vi "DDS.vi"() -> ()   [LabVIEW 2021]
uses:
  <vilib>/RTI DDS Toolkit/Types/RTI DDS Advanced Writer Configuration.ctl
  <vilib>/RTI DDS Toolkit/Types/RTI DDS Advanced Reader Configuration.ctl
  <vilib>/Platform/TimedLoop/XDataNode/timing_clust.ctl
  <vilib>/Platform/TimedLoop/XDataNode/nitl_modes.ctl
  <vilib>/Platform/TimedLoop/XDataNode/wakeup.ctl
  <vilib>/RTI DDS Toolkit/VIs/AdvancedCreateWriter_NumI32.vi
  <vilib>/RTI DDS Toolkit/VIs/Write_NumI32.vi
  <vilib>/Platform/TimedLoop/XDataNode/XDataNode.xnode
  <vilib>/RTI DDS Toolkit/VIs/Read_NumI32.vi
  <vilib>/RTI DDS Toolkit/VIs/AdvancedCreateReader_NumI32.vi
  <vilib>/RTI DDS Toolkit/Library/LVDDS_library.lvlib
  <vilib>/Platform/TimedLoop/XDataNode/XDNodeRunTimeDep.lvlib
panel:
  in  "Advanced Reader Configuration":T1={"typeName"="std_msgs::msg::dds_::Int32_", "keyName"="", "domainParticipantQoSProfile"="", "dataReaderQoSProfile"="", "forceArrayMapping?"=FALSE, "forceExclusiveReader?"=FALSE, "forceRead? (only ExclusiveReader)"=FALSE, "forceUnboundedString?"=FALSE}
  in  "error in (no error)":errorcluster
  in  "Advanced Writer Configuration":T2={"typeName"="std_msgs::msg::dds_::Int32_", "keyName"="", "domainParticipantQoSProfile"="", "dataWriterQoSProfile"="", "forceArrayMapping?"=FALSE, "forceUnboundedString?"=FALSE}
  in  "stop":bool
  # "DDS Communication"
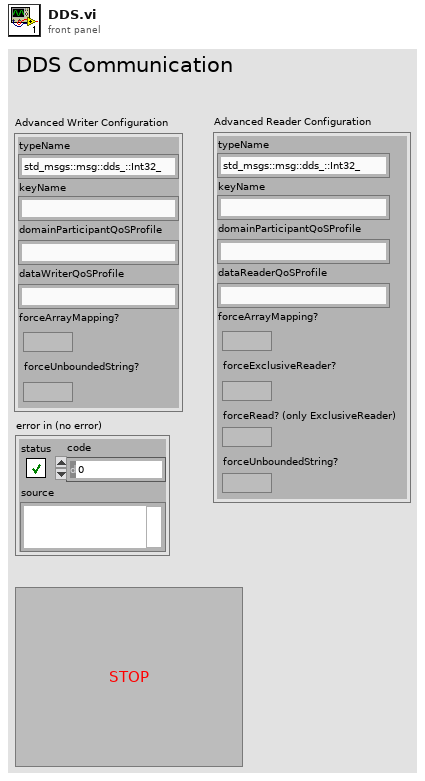
[diagram p1: front panel]
types:
  T1 = typedef "LVDDS_library.lvlib/RTI DDS Advanced Reader Configuration.ctl" = cluster{"typeName":string, "keyName":string, "domainParticipantQoSProfile":string, "dataReaderQoSProfile":string, "forceArrayMapping?":bool, "forceExclusiveReader?":bool, "forceRead? (only ExclusiveReader)":bool, "forceUnboundedString?":bool}
  T2 = typedef "LVDDS_library.lvlib/RTI DDS Advanced Writer Configuration.ctl" = cluster{"typeName":string, "keyName":string, "domainParticipantQoSProfile":string, "dataWriterQoSProfile":string, "forceArrayMapping?":bool, "forceUnboundedString?":bool}
  T3 = typedef "XDNodeRunTimeDep.lvlib/timing_clust.ctl" = cluster{"Expected End [f-1]":u64, "Actual End [f-1]":u64, "Finished Late? [f-1]":bool, "Expected End [i-1]":u64, "Actual End [i-1]":u64, "Finished Late? [i-1]":bool, "Expected Start [i]":u64, "Actual Start [i]":u64, "Expected Start [f]":u64, "Actual Start [f]":u64, "Source Name":string, "Structure Name":string, "Period":i64, "Deadline":i64, "Offset":i64, "Start":i64, "Priority":i32, "Timeout":i32, "Mode":T4, "Wakeup Reason":T5, "Error":errorcluster, "Source Type":string, "Secondary Source Type":string, "Global End Time":u64, "Global Start Time":u64, "Frame Duration":u64, "Iteration Duration":u64, "Assigned CPU":i32, "I/O Scan Engine Mode":u32}
  T4 = typedef "XDNodeRunTimeDep.lvlib/nitl_modes.ctl" = enum32{"No Change", "Process missed periods, maintain original phase", "Discard missed periods, maintain original phase", "Process missed periods, ignore original phase", "Discard missed periods, ignore original phase"}
  T5 = typedef "XDNodeRunTimeDep.lvlib/wakeup.ctl" = enum32{"Normal", "Aborted", "Asynchronous wakeup", "Timing source error", "Timed loop error", "Timeout"}
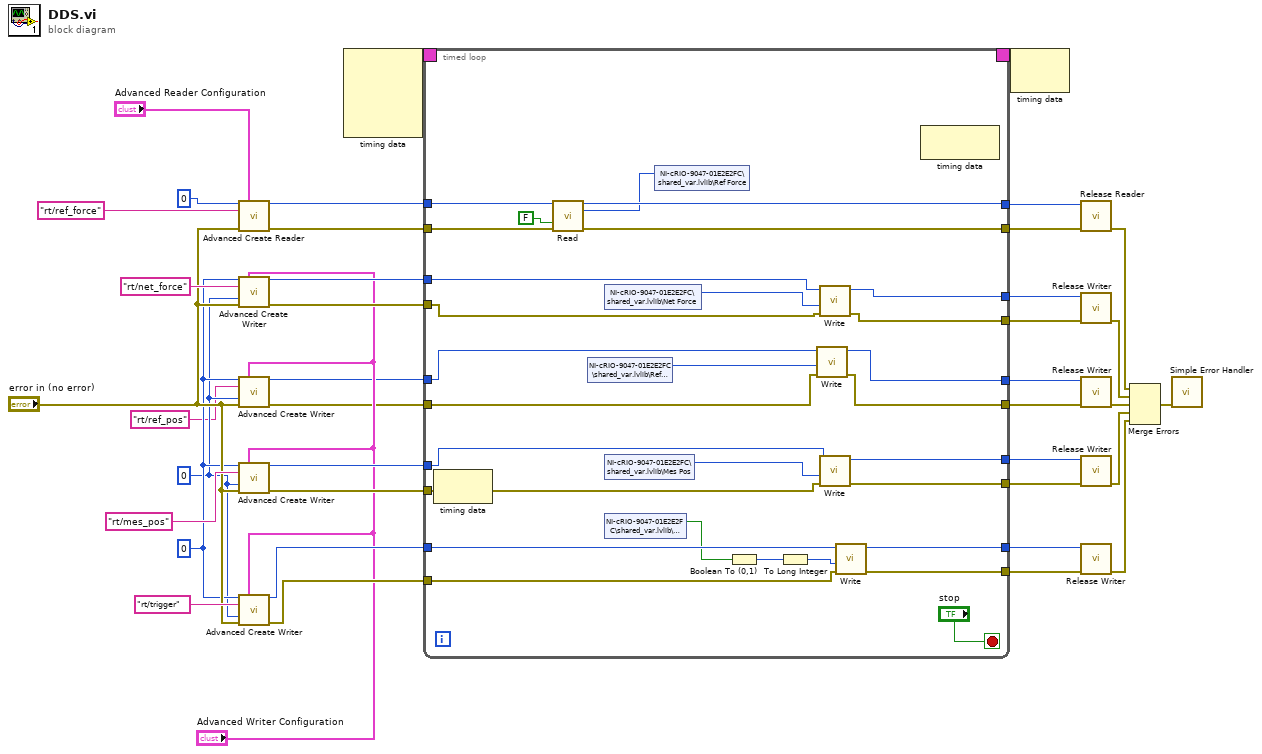
[diagram p0: block diagram]
diagram:
  w9 = 0 ("Data Type")
  w10 = u32 0 ("Domain Id")
  n1 = call-poly <vilib>:"Advanced Create Reader.vi"("Domain Id"=u32 0, "Advanced Reader Configuration"="Advanced Reader Configuration", "Topic Name"="rt/ref_force", "error in (no error)"="error in (no error)") -> ("DDS Object Ref"=w16:u64, "error out"=w17:errorcluster)  [unwired: 10 in]
  n2 = call-poly <vilib>:"Advanced Create Writer.vi"("Domain Id"=w10, "Advanced Writer Configuration"="Advanced Writer Configuration", "Topic Name"="rt/net_force", "Data Type"=w9, "error in (no error)"="error in (no error)") -> ("DDS Object Ref"=w31:u64, "error out"=w30:errorcluster)  [unwired: 9 in]
  n3 = call-poly <vilib>:"Advanced Create Writer.vi"("Domain Id"=w10, "Advanced Writer Configuration"="Advanced Writer Configuration", "Topic Name"="rt/ref_pos", "Data Type"=w9, "error in (no error)"="error in (no error)") -> ("DDS Object Ref"=w7:u64, "error out"=w8:errorcluster)  [unwired: 9 in]
  n4 = call-poly <vilib>:"Advanced Create Writer.vi"("Domain Id"=w10, "Advanced Writer Configuration"="Advanced Writer Configuration", "Topic Name"="rt/mes_pos", "Data Type"=w9, "error in (no error)"="error in (no error)") -> ("DDS Object Ref"=w38:u64, "error out"=w37:errorcluster)  [unwired: 9 in]
  n5 = call-poly <vilib>:"Advanced Create Writer.vi"("Domain Id"=w10, "Advanced Writer Configuration"="Advanced Writer Configuration", "Topic Name"="rt/trigger", "Data Type"=w9, "error in (no error)"="error in (no error)") -> ("DDS Object Ref"=w23:u64, "error out"=w24:errorcluster)  [unwired: 9 in]
  n6 = node-c288() -> (w35:T3)  [unwired: 4 in]
  n7 = timed-loop {
    timing: w35 -> [_]
    timing-out: [_] -> w34
    tunnel: w38 -> [w68]
    tunnel: w37 -> [w67]
    tunnel: [w66] -> w33
    tunnel: [w65] -> w32
    tunnel: w31 -> [w60]
    tunnel: w30 -> [w61]
    tunnel: [w64] -> w29
    tunnel: [w63] -> w28
    tunnel: w24 -> [w59]
    tunnel: w23 -> [w58]
    tunnel: [w57] -> w22
    tunnel: [w56] -> w21
    tunnel: w17 -> [w54]
    tunnel: w16 -> [w53]
    tunnel: [w52] -> w15
    tunnel: [w51] -> w14
    tunnel: w8 -> [w46]
    tunnel: w7 -> [w42]
    tunnel: [w45] -> w6
    tunnel: [w44] -> w5
    stop <- "stop" stop-if-true
    n8 = node-c288() -> ()  [unwired: 1 in, 1 out]
    n9 = call-poly <vilib>:"Read.vi"("DDS Object Ref in"=w53, "Only New Samples"=FALSE, "error in (no error)"=w54) -> ("DDS Object Ref out"=w52:u64, "Data"=w50:i32, "error out"=w51:errorcluster)  [unwired: 8 in, 2 out]
    n10 = shared-variable "NI-cRIO-9047-01E2E2FC\\shared_var.lvlib\\Ref Pos"() -> (w43:i32)  [unwired: 1 in, 1 out]
    n11 = shared-variable "NI-cRIO-9047-01E2E2FC\\shared_var.lvlib\\Net Force"() -> (w40:i32)  [unwired: 1 in, 1 out]
    n12 = shared-variable "NI-cRIO-9047-01E2E2FC\\shared_var.lvlib\\Mes Pos"() -> (w41:i32)  [unwired: 1 in, 1 out]
    n13 = shared-variable "NI-cRIO-9047-01E2E2FC\\shared_var.lvlib\\Trigger"() -> (w49:bool)  [unwired: 1 in, 1 out]
    n14 = shared-variable "NI-cRIO-9047-01E2E2FC\\shared_var.lvlib\\Ref Force"(w50) -> ()  [unwired: 1 in, 1 out]
    n15 = Boolean To (0,1)(Boolean=w49) -> (0, 1=w48:i16)
    n16 = To Long Integer(number=w48) -> (32bit integer=w47:i32)
    n17 = call-poly <vilib>:"Write.vi"("error in (no error)"=w46, "Data"=w43, "DDS Object Ref in"=w42) -> ("error out"=w45:errorcluster, "DDS Object Ref out"=w44:u64)  [unwired: 7 in]
    n18 = call-poly <vilib>:"Write.vi"("error in (no error)"=w61, "Data"=w40, "DDS Object Ref in"=w60) -> ("error out"=w63:errorcluster, "DDS Object Ref out"=w64:u64)  [unwired: 7 in]
    n19 = call-poly <vilib>:"Write.vi"("error in (no error)"=w67, "Data"=w41, "DDS Object Ref in"=w68) -> ("error out"=w65:errorcluster, "DDS Object Ref out"=w66:u64)  [unwired: 7 in]
    n20 = call-poly <vilib>:"Write.vi"("error in (no error)"=w59, "Data"=w47, "DDS Object Ref in"=w58) -> ("error out"=w56:errorcluster, "DDS Object Ref out"=w57:u64)  [unwired: 7 in]
    n21 = node-c288() -> ()  [unwired: 1 in, 1 out]
  }
  n22 = node-c288(w34) -> ()  [unwired: 1 out]
  n23 = call <vilib>:"Release Reader.vi"("error in (no error)"=w14, "DDS Object Ref"=w15) -> ("error out"=w1:errorcluster)  [unwired: 9 in]
  n24 = call <vilib>:"Release Writer.vi"("error in (no error)"=w28, "DDS Object Ref"=w29) -> ("error out"=w4:errorcluster)  [unwired: 9 in]
  n25 = call <vilib>:"Release Writer.vi"("error in (no error)"=w6, "DDS Object Ref"=w5) -> ("error out"=w3:errorcluster)  [unwired: 9 in]
  n26 = call <vilib>:"Release Writer.vi"("error in (no error)"=w32, "DDS Object Ref"=w33) -> ("error out"=w27:errorcluster)  [unwired: 9 in]
  n27 = call <vilib>:"Release Writer.vi"("error in (no error)"=w21, "DDS Object Ref"=w22) -> ("error out"=w13:errorcluster)  [unwired: 9 in]
  n28 = Merge Errors(w1, w4, w3, w27, w13) -> (w26:errorcluster)
  n29 = call <vilib>:"Simple Error Handler.vi"("error in (no error)"=w26) -> ()  [unwired: 4 in, 5 out]
